vi "hidSPD Read Report.vi"(8 "error in (no error)":errorcluster, 11 "spdDevSession in":T1) -> (0 "error out":errorcluster, 1 "data":i32[](array[numeric]), 2 "cmd":i32, 3 "spdDevSession out":T1)   [LabVIEW 2018, in "hidSPDLibForLabView.lvlib"]
uses:
  hidSPDLibForLabView.lvlib
  hidSPD Controls/hidSPD Device Session.ctl
  <vilib>/Utility/error.llb/Error Cluster From Error Code.vi
  <vilib>/ErrorRing/Error Ring.xnode
  hidSPD DLL files/libSPD.dll
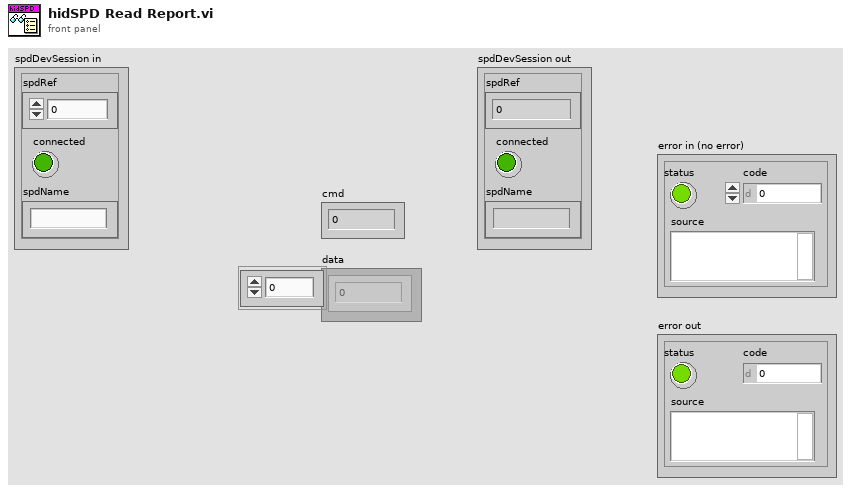
[diagram p1: front panel]
types:
  T1 = typedef "hidSPDLibForLabView.lvlib/hidSPD Device Session.ctl" = cluster{"spdRef":u64, "connected":bool, "spdName":string}
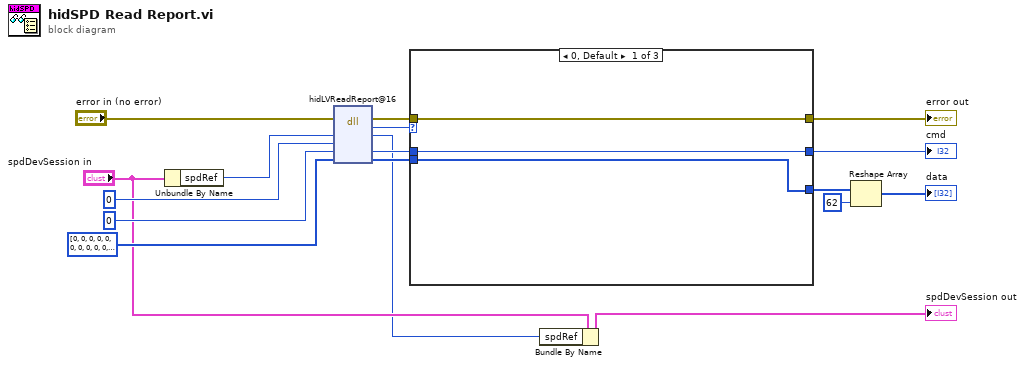
[diagram p0: block diagram]
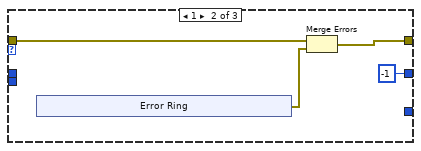
[diagram p2: hidden frame]
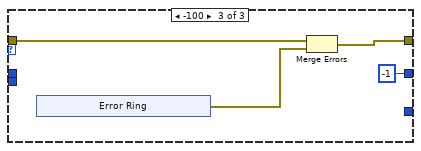
[diagram p3: hidden frame]
diagram:
  n1 = Unbundle By Name("spdDevSession in") -> ("spdRef"=w8:u64)
  n2 = dll-call lib="D:/NextCloud/SPD/hidSPDLibForLabView/hidSPD DLL files/libSPD.dll" fn="hidLVReadReport@16"(error in="error in (no error)", "spdDeviceHandle"=w8, "id"=0 ("report"), "cmd"=0, "data"=i32[] [0, 0, 0, 0, 0, 0, 0, 0, 0, 0, 0, 0, 0, 0, 0, 0, 0, 0, 0, 0, 0, 0, 0, 0, 0, 0, 0, 0, 0, 0, 0, 0, 0, 0, 0, 0, 0, 0, 0, 0, 0, 0, 0, 0, 0, 0, 0, 0, 0, 0, 0, 0, 0, 0, 0, 0, 0, 0, 0, 0, 0, 0]) -> (error out=w9:errorcluster, "error"=w10:i32, "spdDeviceHandle"=w6:u64, "cmd"=w11:i32, "data"=w12:i32[])  [unwired: 3 in, 1 out]
  n3 = case shown="0, Default" w10 {
    tunnel: [w20 w22 w31] -> w17
    tunnel: w12 -> [w18 _ _]
    tunnel: w11 -> [w19 _ _]
    tunnel: w9 -> [w20 w24 w33]
    tunnel: [w19 -1 ("cmd") -1 ("cmd")] -> w4
    tunnel: [w18 _ _] -> w3
    frame 0, Default {
    }
    frame 1 {
      n4 = xnode "Error Ring"() -> ("error out"=w23:errorcluster)
      n5 = Merge Errors(w24, w23) -> (w22:errorcluster)
    }
    frame -100 {
      n6 = xnode "Error Ring"() -> ("error out"=w32:errorcluster)
      n7 = Merge Errors(w33, w32) -> (w31:errorcluster)
    }
  }
  "error out" <- w17
  "cmd" <- w4
  n8 = Bundle By Name(cluster="spdDevSession in", "spdRef"=w6) -> (→"spdDevSession out":T1)
  n9 = Reshape Array(w3, 62 ("dimension size")) -> (→"data":i32[])
